vi "Main-Page - userevent_QHM.vi"() -> ()   [LabVIEW 2015]
uses:
  <vilib>/Utility/miscctls.llb/LVPointTypeDef.ctl
  0.Main_Control/Control_QHM_Behavior.ctl
  0.Main_Control/Control_QHM_Buttom.ctl
  0.Main_Control/Control_QHM_action_userDataManager.ctl
  0.Main_Control/Control_QHM_action_SystemControl.ctl
  2.0_Function/Function_VISA/Control/Control_Axis Number.ctl
panel:
  in  "使用者帳戶":path=path "D:/全域高斯機 參數/use history"
  in  "參數設定":path=path "D:/全域高斯機 參數/use history"
  out "狀態：":string="可使用"
  out "群組：":string="開發人員"
  in  "原點資訊":path=path "D:/全域高斯機 參數/Original"
  in  "匯入硬體參數":path=path "D:/全域高斯機 參數/use history"
  in  "儲存檔案路徑":path=path "D:/全域高斯機Data"
  in  "匯入圖檔(Setting)":path=path "D:/全域高斯機資料/TAHOE3.png"
  out "狀態：":T1
  in  "離開程式":bool
  out "群組：":T2
  out "帳號：":string="admin"
  in  "關於本系統":bool
  in  "資料管理":bool
  in  "登出/離開":bool
  in  "系統管理選單":bool
  in  "開始":bool
  in  "每日檢測":bool
  # "C:\\Users\\jyun.huang.MINAIK\\Desktop\\四穴雷切\\參數設定\\Data\\參數設定"
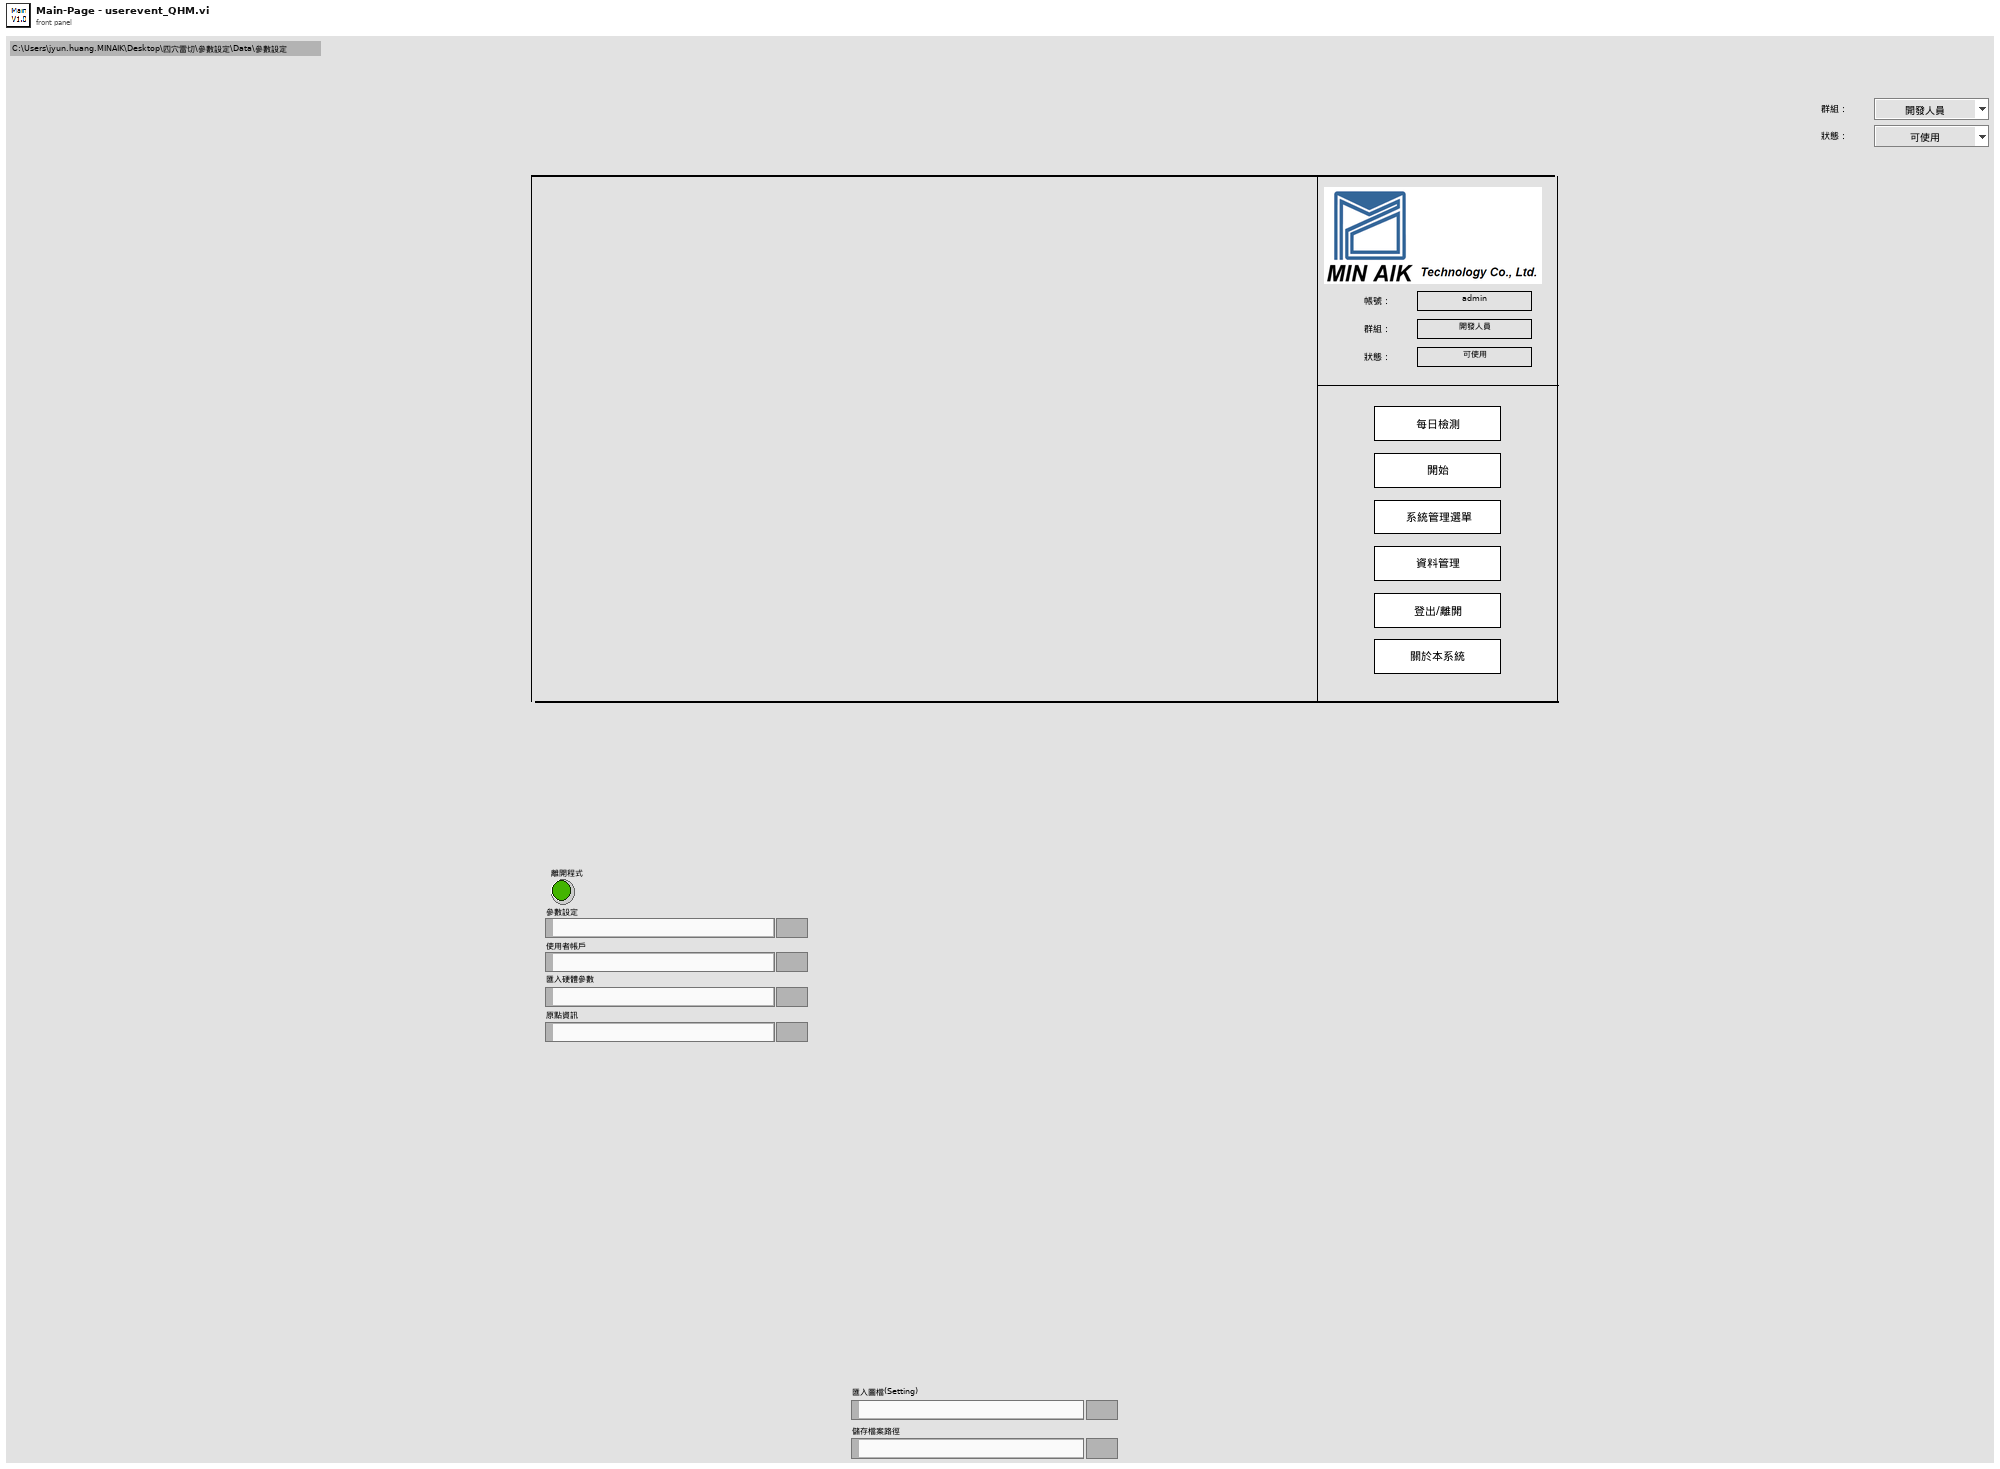
[diagram p1: front panel]
types:
  T1 = typedef "Control_User Accounts_Status.ctl" = enum16{"可使用", "不可使用"}
  T2 = typedef "Control_User account_Permissions.ctl" = enum16{"開發人員", "管理者", "工程師", "作業員"}
  T3 = typedef "Control_QHM_Behavior.ctl" = cluster{string, "動作":enum16{"使用者登入", "系統初始化"}}
  T4 = typedef "LVPointTypeDef.ctl" = cluster{"Horizontal":i16, "Vertical":i16}
  T5 = typedef "Control_Original.ctl" = cluster{"R":dbl, "Y":dbl, "Z":dbl, "Angle":dbl}
  T6 = typedef "Control_軸參數.ctl" = cluster{"Name":string, "VISA In":refnum<visa-resource-name>, "R":dbl, "Y":dbl, "Z":dbl, "θ":dbl, "最大值":dbl, "最小值":dbl, "VISA Data":cluster{"Baud rate":u32, "Data bits":u16, "Parity":enum16{"None", "Odd", "Even", "Mark", "Space"}, "Stop bits":u16, "Flow control":u16}, "Paremeter":T7, "DAQ Paremeter":cluster{"Task In":refnum<k21>, "Physical Channels":tag, "Max Value":dbl, "Min Value":dbl, "Rate":dbl}}
  T7 = typedef "Control_手動測試_軸參數.ctl" = cluster{"Scan speed":T8, "Power":u16, "Angle":dbl, "X":i32, "X":i32, "Xc":i32}
  T8 = typedef "Control_Axis Number.ctl" = u16
  T9 = typedef "Control_Main_All Data.ctl" = enum16{"Initialize", "Set Data", "Get Data"}
  T10 = typedef "Use History.ctl" = enum16{"Initialize", "Set Data", "Get Data", "Idle"}
  T11 = typedef "Control_QHM_Buttom.ctl" = cluster{"DataName":string, "Data":enum16{"每日點檢", "開始", "系統管理選單", "資料管理", "登出/離開", "關於本系統"}}
  T12 = enum16{"每日點檢", "開始", "系統管理選單", "資料管理", "登出/離開", "關於本系統"}
  T13 = typedef "Control_User account_Data.ctl" = cluster{"帳號 :":string, "權限等級：":T2, "建立時間：":string, "修改時間：":string, "到期時間：":string, "狀態：":T1, "期限：":T14, "密碼：":string}
  T14 = typedef "Control_User account_Date.ctl" = enum16{"零天", "一天", "七天", "一個月", "一年", "三年"}
  T15 = typedef "Control_QHM_action_userDataManager.ctl" = cluster{"String":string, "帳號管理":enum16{"登入", "確認狀態", "更新介面", "帳號管理", "登出"}}
  T16 = typedef "Action_Data.ctl" = enum16{"Initialize", "Get Data", "Set Data", "Delete Data", "Idle"}
  T17 = cluster{cluster{"掃描速度":i32, "功率":i32, "切割刀數":dbl, "左/右":string}, cluster{"掃描速度2":i32, "功率2":i32, "切割刀數2":dbl, "左/右":string}, cluster{"掃描速度3":i32, "功率3":i32, "切割刀數3":dbl, "左/右":string}, cluster{"掃描速度4":i32, "功率4":i32, "切割刀數4":dbl, "左/右":string}, cluster{"掃描速度5":i32, "功率5":i32, "切割刀數5":dbl, "左/右":string}}
  T18 = typedef "Control_QHM_action_SystemControl.ctl" = cluster{"String":string, "系統":enum16{"關機", "等待", "回到作業系統"}}
  T19 = enum16{"All Enable", "All Disable", "Port Enable", "Port Disable"}
  T20 = cluster{"掃描速度5":i32, "功率5":i32, "切割刀數5":dbl, "左/右":string}
  T21 = typedef "Control_Bounce Window_Main_System Configuration.ctl" = enum16{"帳號管理", "手動操作", "機器參數設定", "離開", "等待"}
  T22 = typedef "Control_Bounce Window_Main_Data Management.ctl" = enum16{"量測參數設定", "操作履歷", "數據回顧", "離開", "等待"}
  T23 = typedef "Control_Bounce Window_Main_Log On-Exit.ctl" = enum16{"回到作業系統", "關機", "使用者登出", "離開", "等待"}
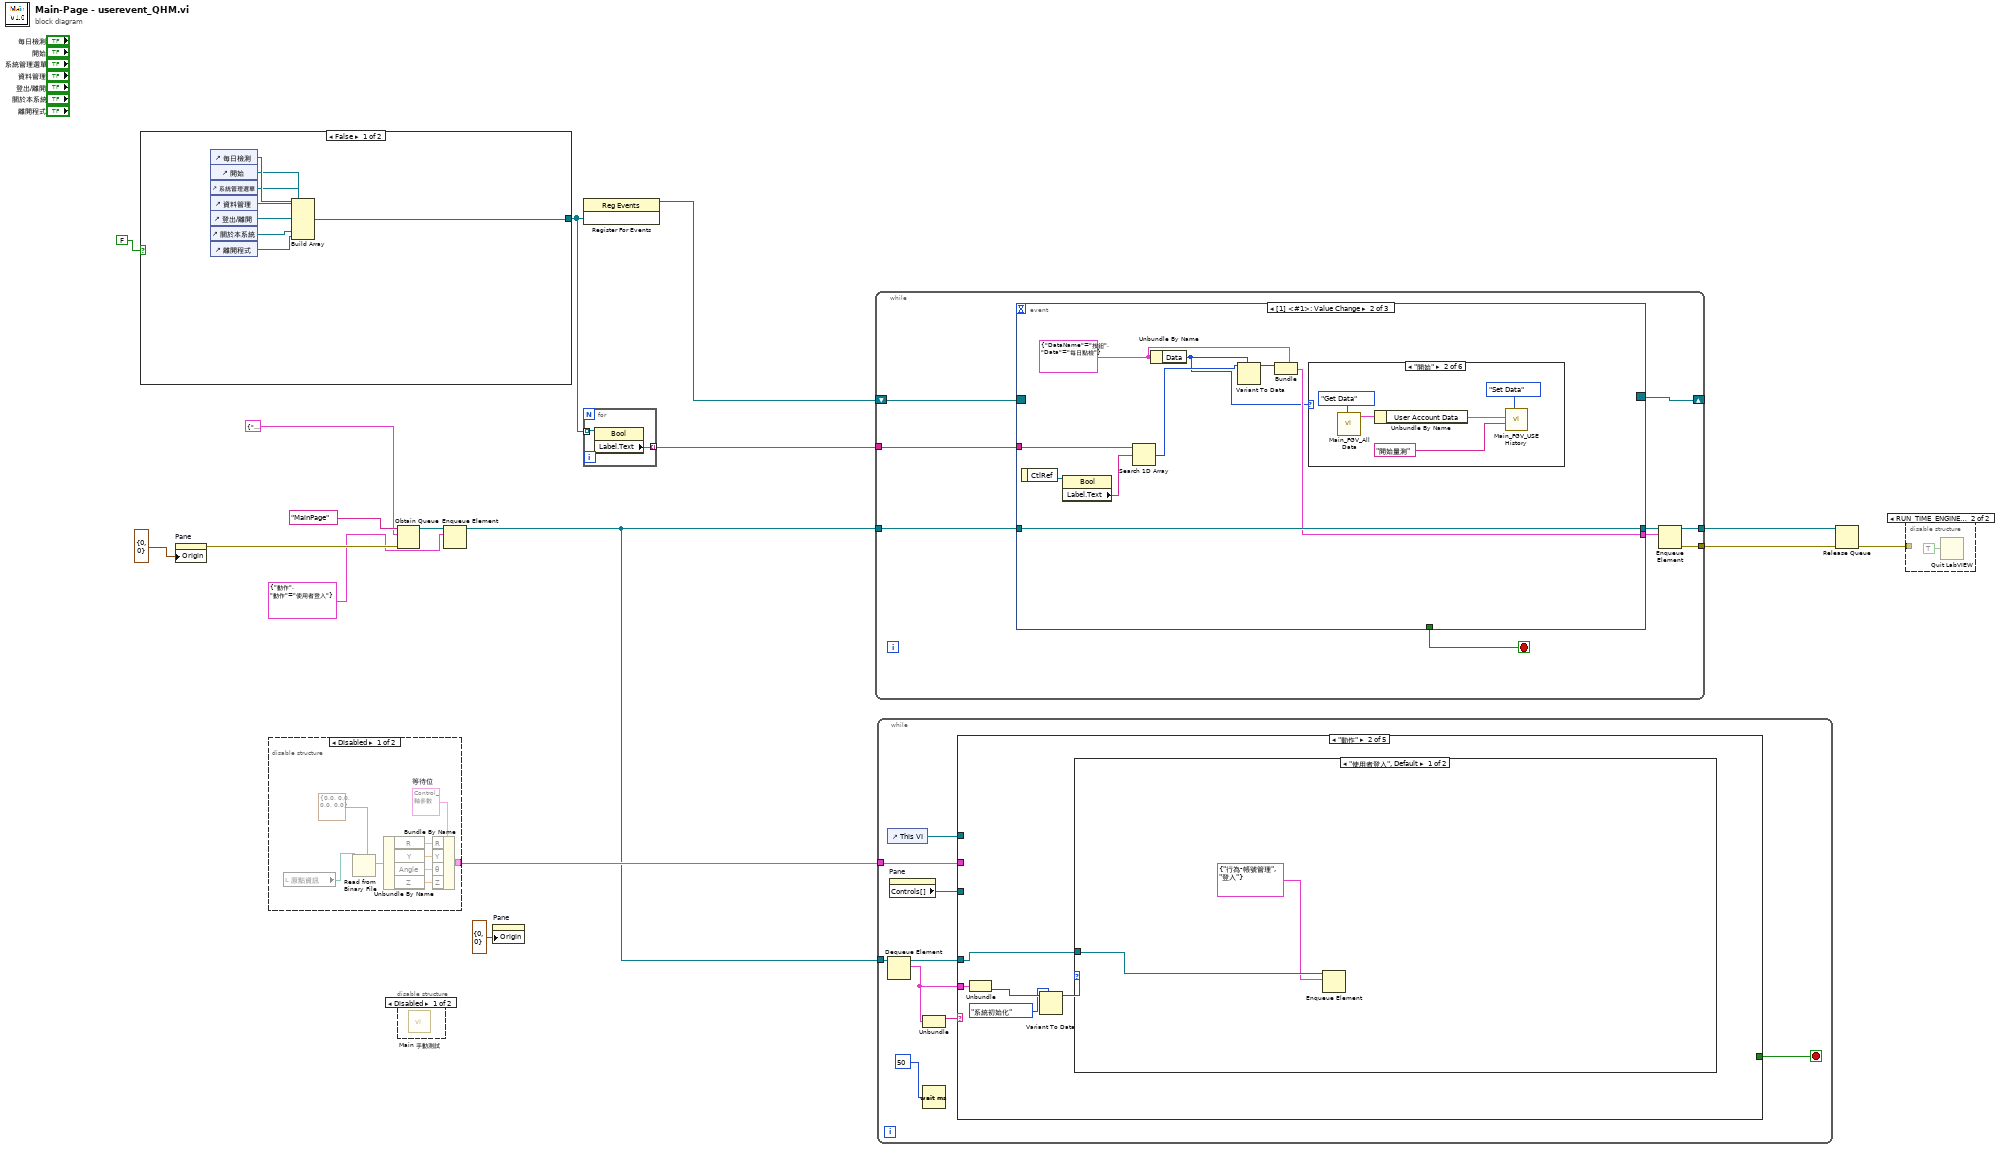
[diagram p0: block diagram]
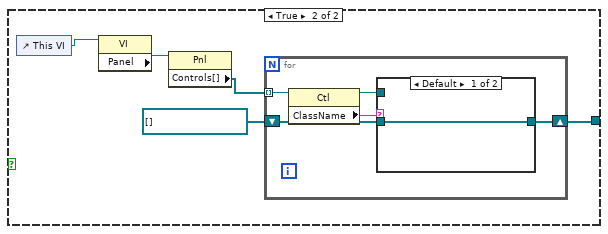
[diagram p2: hidden frame]
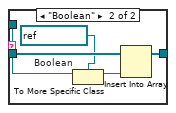
[diagram p3: hidden frame]
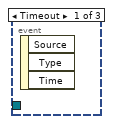
[diagram p4: hidden frame]
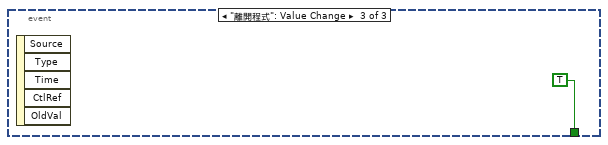
[diagram p10: hidden frame]
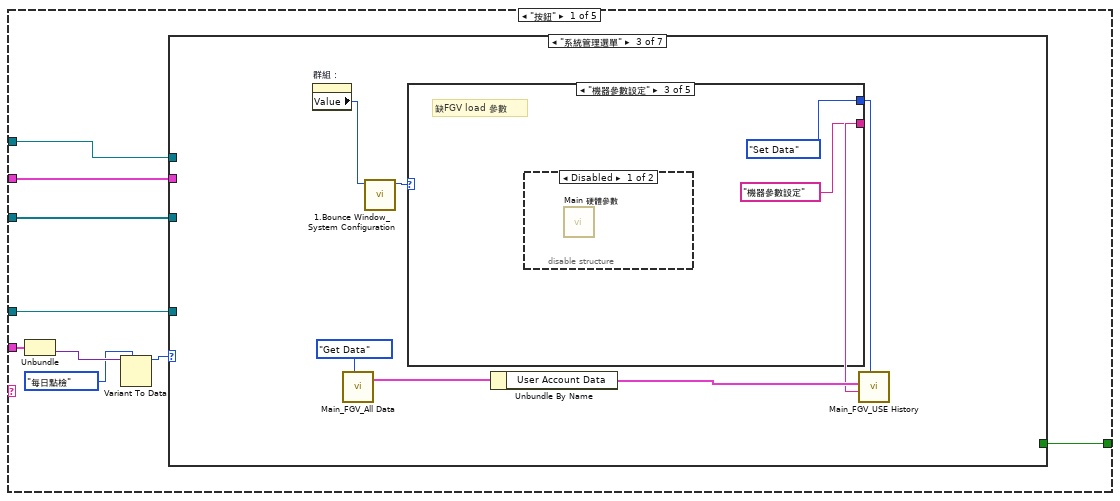
[diagram p14: hidden frame]
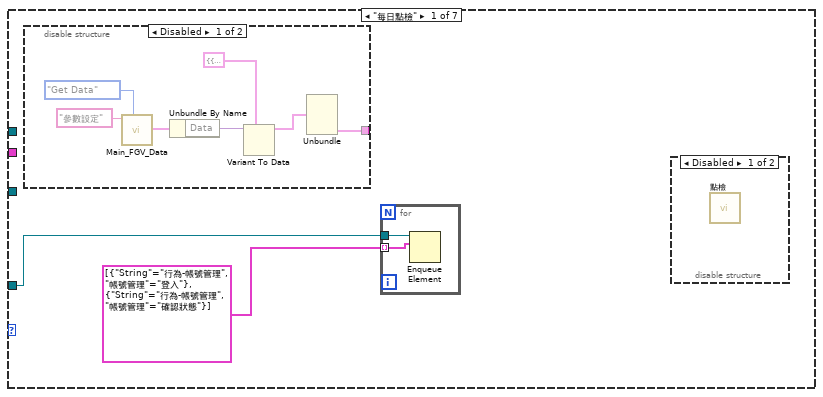
[diagram p15: hidden frame]
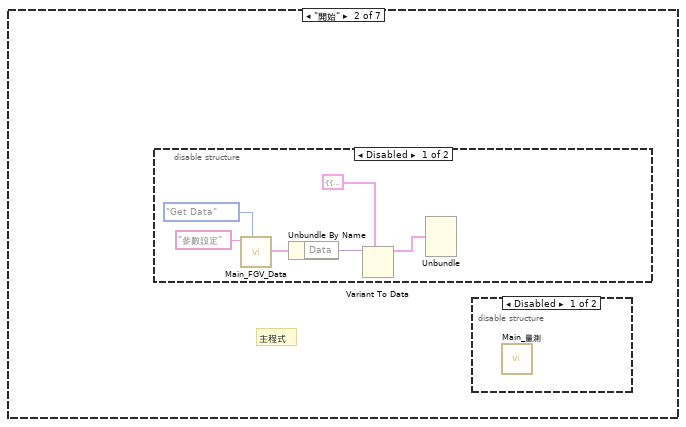
[diagram p18: hidden frame]
diagram:
  n1 = case shown="False" FALSE {
    tunnel: [w17 w25] -> w6
    frame False {
      n2 = control-ref of="每日檢測"() -> (w24:refnum<vi>)
      n3 = control-ref of="開始"() -> (w23:refnum<vi>)
      n4 = control-ref of="系統管理選單"() -> (w22:refnum<vi>)
      n5 = control-ref of="資料管理"() -> (w21:refnum<vi>)
      n6 = control-ref of="登出/離開"() -> (w20:refnum<vi>)
      n7 = control-ref of="關於本系統"() -> (w19:refnum<vi>)
      n8 = control-ref of="離開程式"() -> (w18:refnum<vi>)
      n9 = Build Array(w24, w23, w22, w21, w20, w19, w18) -> (w17:refnum<vi>[])
    }
    frame True {
      n10 = control-ref of="This VI"() -> (w29:refnum<vi>)
      n11 = property class="VI"(reference=w29) -> ("Panel"=w28:refnum<vi>)  [unwired: 1 in, 2 out]
      n12 = property class="Pnl"(reference=w28) -> ("Controls[]"=w27:refnum<vi>[])  [unwired: 1 in, 2 out]
      n13 = for {
        tunnel: w27 -> [w32] mode=indexing
        shift-right: [w31] -> w25
        shift-left: refnum<vi>[] [] -> [w33]
        n14 = property class="Ctl"(reference=w32) -> ("ClassName"=w30:string)  [unwired: 1 in, 2 out]
        n15 = case shown="Default" w30 {
          tunnel: w33 -> [w34 w39]
          tunnel: w32 -> [_ w38]
          tunnel: [w34 w36] -> w31
          frame Default {
          }
          frame "Boolean" {
            w37 = refnum<vi> refnum  # Boolean
            n16 = To More Specific Class(target class=w37, reference=w38) -> (specific class reference=w35:refnum<vi>)  [unwired: 1 in, 1 out]
            n17 = Insert Into Array(array=w39, new element=w35) -> (w36:refnum<vi>[])  [unwired: 1 in]
          }
        }
      }
    }
  }
  n18 = property on="Pane" class="Pane"("Origin"=T4 {"Horizontal"=0, "Vertical"=0}) -> (error out=w11:errorcluster)  [unwired: 2 in, 1 out]
  n19 = disable-structure shown="Disabled" {
    disable-tunnel: [w41 _] -> w14
    frame Disabled {
      w42 = T6 {"Name"="", "VISA In"="COM2", "R"=40.8, "Y"=12.9, "Z"=0.0, "θ"=87.62, "最大值"=0.0, "最小值"=0.0, "VISA Data"={"Baud rate"=115200, "Data bits"=8, "Parity"=enum."Even", "Stop bits"=10, "Flow control"=0}, "Paremeter"={"Scan speed"=4, "Power"=2, "Angle"=0.0, "X"=9000, "X"=60000, "Xc"=60000}, "DAQ Paremeter"={"Task In"="CalibrationTest", "Physical Channels"="Dev1/ai0", "Max Value"=10.0, "Min Value"=-10.0, "Rate"=1000.0}}  # 等待位
      n20 = local read "原點資訊"() -> (w40:path)
      n21 = Read from Binary File(5:T5 {"R"=0.0, "Y"=0.0, "Z"=0.0, "Angle"=0.0} ("治具原點"), 11:w40) -> (2:w47:T5)  [unwired: 4 in, 3 out]
      n22 = Unbundle By Name(w47) -> ("R"=w46:dbl, "Y"=w45:dbl, "Angle"=w44:dbl, "Z"=w43:dbl)
      n23 = Bundle By Name(cluster=w42, "R"=w46, "Y"=w45, "θ"=w44, "Z"=w43) -> (w41:T6)
    }
    frame Enabled {
    }
  }
  n24 = Obtain Queue(name (unnamed)="MainPage", element data type=cluster{string, variant} {"", variant}, error in (no error)=w11) -> (queue out=w12:refnum<queue>)  [unwired: 2 in, 2 out]
  n25 = disable-structure shown="Disabled" {
    frame Disabled {
      n26 = call "Main 手動測試.vi"() -> ()  [unwired: 12 in]
    }
    frame Enabled {
    }
  }
  n27 = Enqueue Element(queue=w12, element=T3 {"動作", "動作"=enum."使用者登入"} ("output cluster")) -> (queue out=w1:refnum<queue>)  [unwired: 2 in, 2 out]
  n28 = property on="Pane" class="Pane"("Origin"=T4 {"Horizontal"=0, "Vertical"=0}) -> ()  [unwired: 2 in, 2 out]
  n29 = register-events(w6) -> (reference out=w10:refnum<event-registration>)  [unwired: 2 in, 1 out]
  n30 = for {
    tunnel: w6 -> [w50] mode=indexing
    tunnel: [w49] -> w5 mode=indexing
    n31 = property class="Bool"(reference=w50) -> ("Label.Text"=w49:string)  [unwired: 1 in, 2 out]
  }
  n32 = while {
    shift-right: [w58] -> _
    shift-left: w10 -> [w59]
    tunnel: w5 -> [w57]
    tunnel: w1 -> [w55]
    tunnel: [w54] -> w8
    tunnel: [w53] -> w7
    stop <- w52 stop-if-true
    n33 = event shown="[1] <#1>: Value Change" {
      selector: w59 -> [_ _ _]
      dyn-events: [_ _ _] -> w58
      timeout: _ -> [_ _ _]
      tunnel: w57 -> [_ w68 _]
      tunnel: [_ w66 _] -> w56
      tunnel: w55 -> [_ w66 _]
      tunnel: [_ w61 _] -> w51
      tunnel: [_ _ TRUE] -> w52
      event Timeout {
        n34 = event-data() -> ()  [unwired: 1 in, 3 out]
      }
      event Value Change {
        w63 = T11 {"DataName"="按鈕", "Data"=enum."每日點檢"} ("output cluster")
        n35 = event-data() -> ("CtlRef"=w65:refnum<vi>)  [unwired: 1 in]
        n36 = property class="Bool"(reference=w65) -> ("Label.Text"=w67:string)  [unwired: 1 in, 2 out]
        n37 = Search 1D Array(1D array=w68, element=w67) -> (index of element=w64:i32)  [unwired: 1 in]
        n38 = Unbundle By Name(w63) -> ("Data"=w60:T12)
        n39 = Variant To Data(type=w60, Variant=w64) -> (data=w62:T12)  [unwired: 1 in, 1 out]
        n40 = Bundle(cluster=w63, "Data"=w62) -> (w61:T11)  [unwired: 1 in]
        n41 = case shown="\"開始\"" w60 {
          frame "每日點檢", Default {
          }
          frame "開始" {
            n42 = call "Main_FGV_All Data.vi"("Data_Action"=Control_Main_All_Data."Get Data") -> ("All Data Out"=w73:cluster{"User Account Data":T13})  [unwired: 9 in, 1 out]
            n43 = Unbundle By Name(w73) -> ("User Account Data"=w70:T13)
            n44 = call "Main_FGV_USE History.vi"("Use Action"=Use_History."Set Data", "Event"="開始量測", "User Account Data"=w70) -> ()  [unwired: 8 in, 1 out]
          }
          frame "系統管理選單" {
          }
          frame "資料管理" {
          }
          frame "登出/離開" {
          }
          frame "關於本系統" {
          }
        }
      }
      event "離開程式": Value Change {
        n45 = event-data() -> ()  [unwired: 1 in, 5 out]
      }
    }
    n46 = Enqueue Element(queue=w56, element=w51) -> (queue out=w54:refnum<queue>, error out=w53:errorcluster)  [unwired: 2 in, 1 out]
  }
  n47 = while {
    tunnel: w1 -> [w79]
    tunnel: w14 -> [w80]
    stop <- w83 stop-if-true
    n48 = control-ref of="This VI"() -> (w82:refnum<vi>)
    n49 = Dequeue Element(queue=w79) -> (queue out=w78:refnum<queue>, element=w77:cluster{string, variant})  [unwired: 2 in, 2 out]
    n50 = property on="Pane" class="Pane"() -> ("Controls[]"=w81:refnum<vi>[])  [unwired: 2 in, 2 out]
    n51 = Unbundle(w77) -> (w76:string)  [unwired: 1 out]
    n52 = Wait (ms)(milliseconds to wait=u32 50) -> ()  [unwired: 1 out]
    n53 = case shown="\"動作\"" w76 {
      tunnel: [w92 _ w197 _ _] -> w83
      tunnel: w82 -> [w91 _ _ w214 _]
      tunnel: w81 -> [w90 _ _ w212 _]
      tunnel: w80 -> [w89 _ _ _ _]
      tunnel: w78 -> [w88 w166 _ w213 _]
      tunnel: w77 -> [w87 w169 w201 w210 _]
      frame "按鈕" {
        n54 = Unbundle(w87) -> (w86:variant)  [unwired: 1 out]
        n55 = Variant To Data(type=T12."每日點檢" ("按鈕"), Variant=w86) -> (data=w84:T12)  [unwired: 1 in, 1 out]
        n56 = case shown="\"系統管理選單\"" w84 {
          tunnel: [_ _ _ _ _ _ FALSE] -> w92
          tunnel: w88 -> [w94 _ _ _ w143 _ _]
          tunnel: w91 -> [_ _ _ _ _ _ _]
          tunnel: w90 -> [_ _ _ _ _ _ _]
          tunnel: w89 -> [_ _ _ w128 _ _ _]
          frame "每日點檢" {
            n57 = disable-structure shown="Disabled" {
              disable-tunnel: [w95 _] -> _
              frame Disabled {
                n58 = call "Main_FGV_Data.vi"("Action_Data"=Action_Data."Get Data", "Data name"="參數設定") -> ("Data  Out"=w99:cluster{"Data name":string, "Data":variant})  [unwired: 8 in, 1 out]
                n59 = Unbundle By Name(w99) -> ("Data"=w98:variant)
                n60 = Variant To Data(type=T17 {{"掃描速度"=0, "功率"=0, "切割刀數"=0.0, "左/右"=""}, {"掃描速度2"=0, "功率2"=0, "切割刀數2"=0.0, "左/右"=""}, {"掃描速度3"=0, "功率3"=0, "切割刀數3"=0.0, "左/右"=""}, {"掃描速度4"=0, "功率4"=0, "切割刀數4"=0.0, "左/右"=""}, {"掃描速度5"=0, "功率5"=0, "切割刀數5"=0.0, "左/右"=""}} ("output cluster"), Variant=w98) -> (data=w97:T17)  [unwired: 1 in, 1 out]
                n61 = Unbundle(w97) -> (w95:T20)  [unwired: 4 out]
              }
              frame Enabled {
              }
            }
            n62 = for {
              tunnel: w94 -> [w103]
              tunnel: T15[] [{"String"="行為-帳號管理", "帳號管理"=enum."登入"}, {"String"="行為-帳號管理", "帳號管理"=enum."確認狀態"}] -> [w102] mode=indexing
              n63 = Enqueue Element(queue=w103, element=w102) -> ()  [unwired: 2 in, 3 out]
            }
            n64 = disable-structure shown="Disabled" {
              frame Disabled {
                n65 = call "點檢.vi"() -> ()  [unwired: 12 in]
              }
              frame Enabled {
              }
            }
          }
          frame "開始" {
            # "主程式"
            n66 = disable-structure shown="Disabled" {
              frame Disabled {
                n67 = call "Main_FGV_Data.vi"("Action_Data"=Action_Data."Get Data", "Data name"="參數設定") -> ("Data  Out"=w107:cluster{"Data name":string, "Data":variant})  [unwired: 8 in, 1 out]
                n68 = Unbundle By Name(w107) -> ("Data"=w106:variant)
                n69 = Variant To Data(type=T17 {{"掃描速度"=0, "功率"=0, "切割刀數"=0.0, "左/右"=""}, {"掃描速度2"=0, "功率2"=0, "切割刀數2"=0.0, "左/右"=""}, {"掃描速度3"=0, "功率3"=0, "切割刀數3"=0.0, "左/右"=""}, {"掃描速度4"=0, "功率4"=0, "切割刀數4"=0.0, "左/右"=""}, {"掃描速度5"=0, "功率5"=0, "切割刀數5"=0.0, "左/右"=""}} ("output cluster"), Variant=w106) -> (data=w105:T17)  [unwired: 1 in, 1 out]
                n70 = Unbundle(w105) -> ()  [unwired: 5 out]
              }
              frame Enabled {
              }
            }
            n71 = disable-structure shown="Disabled" {
              frame Disabled {
                n72 = call "Main_量測.vi"() -> ()  [unwired: 11 in]
              }
              frame Enabled {
              }
            }
          }
          frame "系統管理選單" {
            n73 = property on="群組：" class="Enum (strict)"() -> ("Value"=w111:T2)  [unwired: 2 in, 2 out]
            n74 = call "Main_FGV_All Data.vi"("Data_Action"=Control_Main_All_Data."Get Data") -> ("All Data Out"=w116:cluster{"User Account Data":T13})  [unwired: 9 in, 1 out]
            n75 = call "1.Bounce Window_System Configuration.vi"("群組："=w111) -> ("系統管理選單"=w110:T21)  [unwired: 10 in]
            n76 = case shown="\"機器參數設定\"" w110 {
              tunnel: ["帳號管理" ("Event") "手動操作" ("Event") "機器參數設定" ("Event") "" ("Event") "" ("Event")] -> w113
              tunnel: [Use_History."Idle" ("Use Action") Use_History."Set Data" ("Use Action") Use_History."Set Data" ("Use Action") Use_History."Idle" ("Use Action") Use_History."Idle" ("Use Action")] -> w114
              frame "帳號管理", Default {
                n77 = local read "使用者帳戶"() -> (w117:path)
                n78 = call "Bounce Window_User Accounts.vi"("User Account Table Path"=w117) -> ()  [unwired: 11 in]
              }
              frame "手動操作" {
                n79 = disable-structure shown="Disabled" {
                  frame Disabled {
                    n80 = call "Setting.vi"() -> ()  [unwired: 11 in]
                  }
                  frame Enabled {
                  }
                }
              }
              frame "機器參數設定" {
                # "缺FGV load 參數"
                n81 = disable-structure shown="Disabled" {
                  frame Disabled {
                    n82 = call "Main 硬體參數.vi"() -> ()  [unwired: 11 in]
                  }
                  frame Enabled {
                  }
                }
              }
              frame "離開" {
              }
              frame "等待" {
              }
            }
            n83 = Unbundle By Name(w116) -> ("User Account Data"=w115:T13)
            n84 = call "Main_FGV_USE History.vi"("Use Action"=w114, "Event"=w113, "User Account Data"=w115) -> ()  [unwired: 8 in, 1 out]
          }
          frame "資料管理" {
            n85 = property on="群組：" class="Enum (strict)"() -> ("Value"=w129:T2)  [unwired: 2 in, 2 out]
            n86 = call "2.Bounce Window_Data Management.vi"("群組："=w129) -> ("資料管理選單"=w130:T22)  [unwired: 10 in]
            n87 = case shown="\"等待\"" w130 {
              tunnel: w128 -> [_ _ _ _]
              tunnel: [Use_History."Set Data" ("Use Action") Use_History."Set Data" ("Use Action") Use_History."Idle" ("Use Action") Use_History."Idle" ("Use Action")] -> w134
              tunnel: ["量測參數設定" ("Event") "操作履歷" ("Event") _ _] -> w135
              frame "量測參數設定", Default {
              }
              frame "操作履歷" {
                n88 = call "使用者紀錄.vi"() -> ()  [unwired: 12 in]
              }
              frame "離開" {
              }
              frame "等待" {
              }
            }
            n89 = call "Main_FGV_All Data.vi"("Data_Action"=Control_Main_All_Data."Get Data") -> ("All Data Out"=w131:cluster{"User Account Data":T13})  [unwired: 9 in, 1 out]
            n90 = Unbundle By Name(w131) -> ("User Account Data"=w133:T13)
            n91 = call "Main_FGV_USE History.vi"("Use Action"=w134, "Event"=w135, "User Account Data"=w133) -> ()  [unwired: 8 in, 1 out]
          }
          frame "登出/離開" {
            n92 = property on="群組：" class="Enum (strict)"() -> ("Value"=w145:T2)  [unwired: 2 in, 2 out]
            n93 = call "Main_FGV_All Data.vi"("Data_Action"=Control_Main_All_Data."Get Data") -> ("All Data Out"=w147:cluster{"User Account Data":T13})  [unwired: 9 in, 1 out]
            n94 = call "3.Bounce Window_Log On&Exit.vi"("群組："=w145) -> ("登出/離開"=w144:T23)  [unwired: 10 in]
            n95 = case shown="\"使用者登出\"" w144 {
              tunnel: [T18 {"String"="行為-系統控制", "系統"=enum."回到作業系統"} ("output cluster") T18 {"String"="行為-系統控制", "系統"=enum."關機"} ("output cluster") T3 {"動作", "動作"=enum."使用者登入"} ("output cluster") T18 {"String"="行為-系統控制", "系統"=enum."等待"} ("output cluster") T18 {"String"="行為-系統控制", "系統"=enum."等待"} ("output cluster")] -> w142
              tunnel: w147 -> [_ _ _ _ _]
              tunnel: [Use_History."Set Data" ("Use Action") Use_History."Set Data" ("Use Action") Use_History."Set Data" ("Use Action") Use_History."Idle" ("Use Action") Use_History."Idle" ("Use Action")] -> w149
              tunnel: ["回到作業系統" "關機" "登出" _ _] -> w150
              frame "回到作業系統", Default {
              }
              frame "關機" {
              }
              frame "使用者登出" {
              }
              frame "離開" {
              }
              frame "等待" {
              }
            }
            n96 = Unbundle By Name(w147) -> ("User Account Data"=w148:T13)
            n97 = call "Main_FGV_USE History.vi"("Use Action"=w149, "Event"=w150, "User Account Data"=w148) -> ()  [unwired: 8 in, 1 out]
            n98 = Enqueue Element(queue=w143, element=w142) -> ()  [unwired: 2 in, 3 out]
          }
          frame "關於本系統" {
            n99 = call "5.Bounce Window_MSG.vi"("MSG In"="版本：1.0\n日期：20160801") -> ()  [unwired: 11 in]
          }
          frame Default {
          }
        }
      }
      frame "動作" {
        n100 = Unbundle(w169) -> (w170:variant)  [unwired: 1 out]
        n101 = Variant To Data(type=enum16{"使用者登入", "系統初始化"}."系統初始化" ("動作"), Variant=w170) -> (data=w167:enum16{"使用者登入", "系統初始化"})  [unwired: 1 in, 1 out]
        n102 = case shown="\"使用者登入\", Default" w167 {
          tunnel: w166 -> [w172 w173]
          frame "使用者登入", Default {
            n103 = Enqueue Element(queue=w172, element=T15 {"String"="行為-帳號管理", "帳號管理"=enum."登入"} ("output cluster")) -> ()  [unwired: 2 in, 3 out]
          }
          frame "系統初始化" {
            n104 = Build Array("參數設定", "使用者帳戶", "匯入硬體參數", "原點資訊") -> (w189:path[])
            n105 = Enqueue Element(queue=w173, element=T3 {"動作", "動作"=enum."使用者登入"} ("output cluster")) -> ()  [unwired: 2 in, 3 out]
            n106 = call "Main_FGV_All Data.vi"("Data_Action"=Control_Main_All_Data."Initialize") -> ()  [unwired: 9 in, 2 out]
            n107 = for {
              tunnel: w189 -> [w196] mode=indexing
              tunnel: [w195] -> w180
              n108 = call "CreatFoldeFile(Deep).vi"("Path"=w196) -> ("error out"=w195:errorcluster)  [unwired: 8 in, 2 out]
            }
            n109 = local read "匯入硬體參數"() -> (w179:path)
            n110 = call "Main_FGV_USE History.vi"("Use Action"=Use_History."Initialize", "匯入硬體參數"=w179) -> ()  [unwired: 9 in, 1 out]
            n111 = local read "參數設定"() -> (w182:path)
            n112 = call "Main_FGV_Data.vi"("Action_Data"=Action_Data."Initialize") -> ("Data Array out"=w181:cluster{"Data name":string, "Data":variant}[])  [unwired: 9 in, 1 out]
            n113 = Read from Binary File(5:w181, 8:w180, 11:w182) -> (0:w177:errorcluster, 2:w176:cluster{"Data name":string, "Data":variant}[])  [unwired: 3 in, 2 out]
            n114 = case shown="Error" w177 {
              tunnel: w176 -> [w190 _]
              tunnel: [w190 cluster{"Data name":string, "Data":variant}[] [] ("Data Array out")] -> w175
              frame No Error {
              }
              frame Error {
              }
            }
            n115 = for {
              tunnel: w175 -> [w192] mode=indexing
              n116 = Unbundle(w192) -> ("Data name"=w193:string)  [unwired: 1 out]
              n117 = call "Main_FGV_Data.vi"("Action_Data"=Action_Data."Set Data", "Data In"=w192, "Data name"=w193) -> ()  [unwired: 7 in, 2 out]
            }
          }
        }
      }
      frame "行為-系統控制" {
        n118 = Unbundle(w201) -> (w200:variant)  [unwired: 1 out]
        n119 = Variant To Data(type=enum16{"關機", "等待", "回到作業系統"}."關機" ("系統"), Variant=w200) -> (data=w198:enum16{"關機", "等待", "回到作業系統"})  [unwired: 1 in, 1 out]
        n120 = case shown="\"等待\"" w198 {
          tunnel: [TRUE _ TRUE] -> w197
          frame "關機", Default {
            n121 = call <vilib>:"System Exec.vi"("run minimized? (F)"=FALSE, "wait until completion? (T)"=TRUE, "command line"="shutdown -s -f -t 00") -> ()  [unwired: 5 in, 4 out]
          }
          frame "等待" {
          }
          frame "回到作業系統" {
            n122 = property on="離開程式" class="Bool (strict)"("Val(Sgnl)"=TRUE ("Value (Signaling)")) -> ()  [unwired: 2 in, 2 out]
          }
        }
      }
      frame "行為-帳號管理" {
        n123 = Unbundle(w210) -> (w211:variant)  [unwired: 1 out]
        n124 = Variant To Data(type=enum16{"登入", "確認狀態", "更新介面", "帳號管理", "登出"}."登入" ("帳號管理"), Variant=w211) -> (data=w208:enum16{"登入", "確認狀態", "更新介面", "帳號管理", "登出"})  [unwired: 1 in, 1 out]
        n125 = case shown="\"確認狀態\"" w208 {
          tunnel: w214 -> [w216 w236 _ _ _]
          tunnel: w212 -> [w215 w235 _ _ _]
          tunnel: w213 -> [_ w234 _ _ _]
          frame "登入", Default {
            n126 = local read "使用者帳戶"() -> (w232:path)
            n127 = call "Main_Fun_Controls Enable.vi"("Controls Action"=T19."All Enable", "Controls In"=w215, "This VI Reference"=w216) -> ()  [unwired: 9 in]
            n128 = call "Main_FGV_All Data.vi"("Data_Action"=Control_Main_All_Data."Get Data") -> ("All Data Out"=w219:cluster{"User Account Data":T13})  [unwired: 9 in, 1 out]
            n129 = call "Bounce Window_Log In.vi"("User Account Table Path"=w232) -> ("User Account Data Out"=w222:T13)  [unwired: 9 in, 1 out]
            n130 = Bundle By Name(cluster=w219, "User Account Data"=w222) -> (w221:cluster{"User Account Data":T13})
            n131 = Unbundle By Name(w222) -> ("帳號 :"=→"帳號：":string, "權限等級："=w229:T2, "狀態："=w231:T1)
            "群組：" <- w229
            "狀態：" <- w231
            n132 = call "Main_FGV_All Data.vi"("Data_Action"=Control_Main_All_Data."Set Data", "All Data In"=w221) -> ()  [unwired: 8 in, 2 out]
            n133 = To Long Integer(number=w229) -> (32bit integer=w228:i32)
            n134 = To Long Integer(number=w231) -> (32bit integer=w230:i32)
            n135 = property on="群組：" class="Enum (strict)"() -> ("Strings []"=w226:string[])  [unwired: 2 in, 2 out]
            n136 = property on="狀態：" class="Enum (strict)"() -> ("Strings []"=w227:string[])  [unwired: 2 in, 2 out]
            n137 = Index Array(array=w226, index=w228) -> (element=→"群組：":string)
            n138 = Index Array(array=w227, index=w230) -> (element=→"狀態：":string)
          }
          frame "確認狀態" {
            n139 = call "Main_FGV_All Data.vi"("Data_Action"=Control_Main_All_Data."Get Data") -> ("All Data Out"=w238:cluster{"User Account Data":T13})  [unwired: 9 in, 1 out]
            n140 = Unbundle By Name(w238) -> ("User Account Data.到期時間："=w240:string, "User Account Data.狀態："=w243:T1, "User Account Data.權限等級："=w244:T2, "User Account Data"=w245:T13)
            n141 = Format Date/Time String(time format string (%c)="%Y/%m/%d") -> (date/time string=w241:string)  [unwired: 2 in]
            n142 = Greater Or Equal?(x=w240, y=w241) -> (x >= y?=w242:bool)
            n143 = case shown="True" w242 {
              tunnel: w234 -> [w248 w255]
              tunnel: w243 -> [_ w256]
              tunnel: [w248 w254] -> w246
              tunnel: [T3 {"動作", "動作"=enum."使用者登入"} ("output cluster") w253] -> w233
              tunnel: w244 -> [_ w252]
              tunnel: w236 -> [_ w251]
              tunnel: w235 -> [_ w250]
              tunnel: w245 -> [_ w249]
              frame False {
              }
              frame True {
                n144 = case shown="\"可使用\", Default" w256 {
                  tunnel: w255 -> [w266 w272]
                  tunnel: [w266 w272] -> w254
                  tunnel: [T18 {"String"="行為-系統控制", "系統"=enum."等待"} ("output cluster") T3 {"動作", "動作"=enum."使用者登入"} ("output cluster")] -> w253
                  tunnel: w252 -> [w265 _]
                  tunnel: w251 -> [w263 _]
                  tunnel: w250 -> [w262 _]
                  tunnel: w249 -> [w259 _]
                  frame "可使用", Default {
                    n145 = case shown="\"開發人員\", Default" w265 {
                      tunnel: [string[] [] ("Control Name Array In") string[] [] ("Control Name Array In") string[] ["系統管理選"] ("Control Name Array In") string[] ["系統管理選單", "資料管理"] ("Control Name Array In")] -> w261
                      frame "開發人員", Default {
                      }
                      frame "管理者" {
                      }
                      frame "工程師" {
                      }
                      frame "作業員" {
                      }
                    }
                    n146 = call "Main_Fun_Controls Enable.vi"("Controls Action"=T19."Port Disable", "Control Name Array In"=w261, "Controls In"=w262, "This VI Reference"=w263) -> ()  [unwired: 8 in]
                    n147 = call "Main_FGV_USE History.vi"("Use Action"=Use_History."Set Data", "Event"="登入", "User Account Data"=w259) -> ()  [unwired: 8 in, 1 out]
                  }
                  frame "不可使用" {
                  }
                }
              }
            }
            n148 = Enqueue Element(queue=w246, element=w233) -> ()  [unwired: 2 in, 3 out]
          }
          frame "更新介面" {
          }
          frame "帳號管理" {
          }
          frame "登出" {
          }
        }
      }
      frame Default {
      }
    }
  }
  n149 = Release Queue(queue=w8, error in (no error)=w7) -> (error out=w4:errorcluster)  [unwired: 1 in, 2 out]
  n150 = disable-structure shown="RUN_TIME_ENGINE==True" {
    disable-tunnel: w4 -> [_ _]
    frame condition #0 (active) {
    }
    frame condition #1 {
      n151 = Quit LabVIEW(quit? (T)=TRUE) -> ()
    }
  }
